vi "Read Sender.vi"(11 "Destroy Self Msg in":refnum<class "Destroy Self Msg.lvclass">) -> (2 "Sender":refnum<class "Sender.lvclass">)   [LabVIEW 2025, in "jettl.lvlib" / "Destroy Self Msg.lvlib" / "Destroy Self Msg.lvclass"]
uses:
  Destroy Self Msg.lvclass
  Destroy Self Msg.lvclass/Destroy Self Msg.ctl
  Sender/Sender/Sender.lvclass
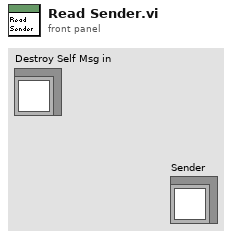
[diagram p1: front panel]
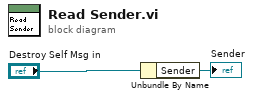
[diagram p0: block diagram]
diagram:
  n1 = Unbundle By Name("Destroy Self Msg in") -> ("Sender"=→"Sender":refnum<class "Sender.lvclass">)
